vi "Config Common.vi"(8 "error in (no error)":errorcluster, 10 "Common Configuration":T1={"Tuner Mode"=0, "Calibration ID"=0, "DUT to Tuner S-parameters"=[[0.0+0.0i, 1.0+0.0i, 1.0+0.0i, 0.0+0.0i]], "Load Termination"=[0.0+0.0i]} {"Tuner Mode" items=["Source", "Load"]}, 11 "iTuner reference in":refnum<k7>) -> (0 "error out":errorcluster, 2 "Primary Frequency (GHz)":dbl, 3 "iTuner reference out":refnum<k7>)   [LabVIEW 2016, in "FocusTuner.lvlib"]
doc: "Configures common settings for load pull using the Focus tuner."
uses:
  FocusTuner.lvlib
  Typedefs/Common Configuration.ctl
  <instrlib>/Focus iTuner Series/Focus iTuner Series.lvlib
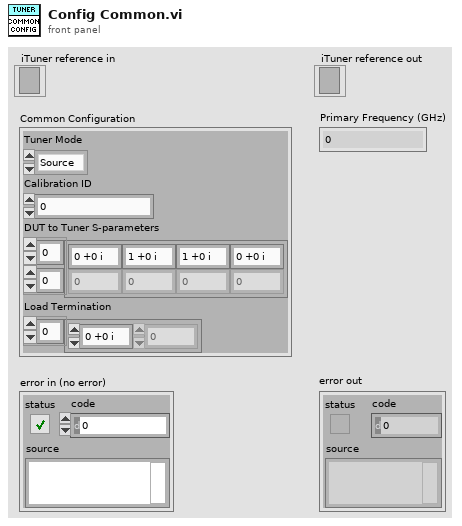
[diagram p1: front panel]
types:
  T1 = typedef "FocusTuner.lvlib/Common Configuration.ctl" = cluster{"Tuner Mode":u16, "Calibration ID":i32, "DUT to Tuner S-parameters":cdb[][], "Load Termination":cdb[]}
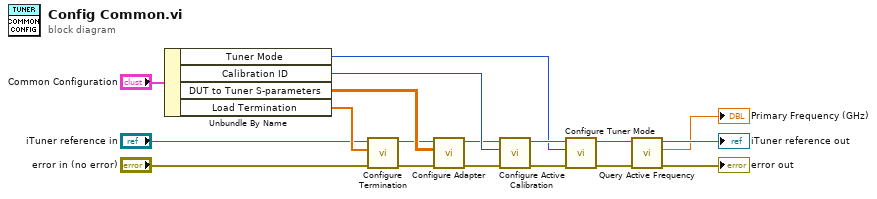
[diagram p0: block diagram]
diagram:
  n1 = Unbundle By Name("Common Configuration") -> ("Tuner Mode"=w15:u16, "Calibration ID"=w14:i32, "DUT to Tuner S-parameters"=w8:cdb[][], "Load Termination"=w7:cdb[])
  n2 = call <instrlib>:"Configure Termination.vi"("error in (no error)"="error in (no error)", "Termination"=w7, "iTuner reference in"="iTuner reference in") -> ("error out"=w2:errorcluster, "iTuner reference out"=w5:refnum<k7>)  [unwired: 7 in]
  n3 = call <instrlib>:"Configure Adapter.vi"("error in (no error)"=w2, "S-parameters"=w8, "iTuner reference in"=w5) -> ("error out"=w1:errorcluster, "iTuner reference out"=w4:refnum<k7>)  [unwired: 7 in]
  n4 = call <instrlib>:"Configure Active Calibration.vi"("error in (no error)"=w1, "Calibration ID (0)"=w14, "iTuner reference in"=w4) -> ("error out"=w16:errorcluster, "iTuner reference out"=w17:refnum<k7>)  [unwired: 7 in]
  n5 = call <instrlib>:"Configure Tuner Mode.vi"("error in (no error)"=w16, "Tuner Mode (0: Source)"=w15, "iTuner reference in"=w17) -> ("error out"=w12:errorcluster, "iTuner reference out"=w13:refnum<k7>)  [unwired: 7 in]
  n6 = call <instrlib>:"Query Active Frequency.vi"("error in (no error)"=w12, "iTuner reference in"=w13) -> ("error out"=→"error out":errorcluster, "Primary Frequency (GHz)"=→"Primary Frequency (GHz)":dbl, "iTuner reference out"=→"iTuner reference out":refnum<k7>)  [unwired: 6 in, 1 out]
